vi "Destroy Timed Average Buffer.vi"(8 "error in (no error)":errorcluster, 11 "Timed Average Buffer":T1) -> (0 "error IO":errorcluster)   [LabVIEW 2015, in "TimedAverageBuffer.lvlib" / "TimedAverageBuffer.lvclass"]
uses:
  TimedAverageBuffer.lvclass
  TimedAverageBuffer Reference.ctl
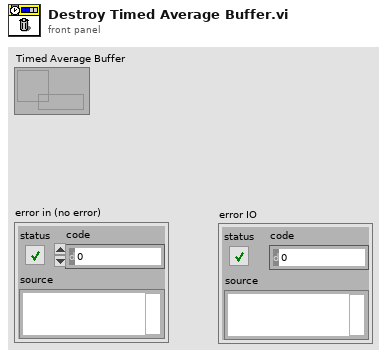
[diagram p1: front panel]
types:
  T1 = typedef "TimedAverageBuffer.lvlib/TimedAverageBuffer.lvclass/TimedAverageBuffer Reference.ctl" = refnum<data-value>
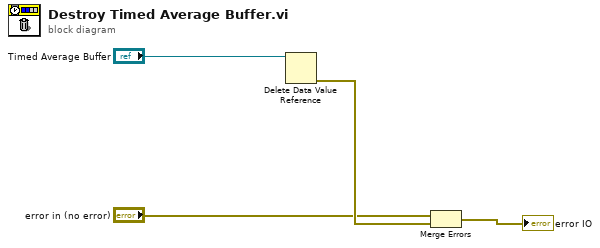
[diagram p0: block diagram]
diagram:
  n1 = Delete Data Value Reference(data value reference="Timed Average Buffer") -> (error out=w3:errorcluster)  [unwired: 1 in, 1 out]
  n2 = Merge Errors("error in (no error)", w3) -> (→"error IO":errorcluster)
